vi "Autonomous Independent.vi"() -> ()   [LabVIEW 2015]
doc: "This VI is called when autonomous begins, and will automatically be terminated when autonomous ends. You can carry out timed or sensor driven robot movement independently without needing to return to the caller."
uses:
  Sprocket/src/Refname/Queues.ctl
  Auto/Auto Modes.ctl
  Sprocket/src/Action/Action Name.ctl
  Sprocket/src/Refname/Refname to String (Queue).vi
  Sprocket/src/Stream/Push Stream.vi
  Sprocket/src/Stream/Release Stream.vi
  Sprocket/lib/Sprocket.lvlib
panel:
  in  "Wedge Drop Power":dbl=0.75
  # "Be sure to right-click and choose Data Operations>>Make Current Value default if you want to save the array values with the VI"
  # "WEDGE"
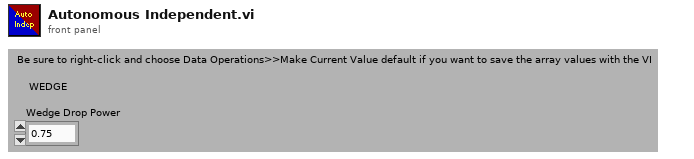
[diagram p1: front panel]
types:
  T1 = typedef "Sprocket.lvlib/Queues.ctl" = enum16{"Input", "Drive", "Collector", "Shifter", "Wedge"}
  T2 = typedef "Auto Modes.ctl" = enum16{"Do Nothing", "Drive Forward", "Cross Low Bar and Stop", "Cross Defense, No Collector", "Cross Ramparts", "Cross Low Bar, Drive to Low Goal, Shoot", "Lower Wedge, Cross Portcullis", "Back n' Forth", "Forward Spin"}
  T3 = typedef "Sprocket.lvlib/Action Name.ctl" = enum16{"No Action", "Drive Train Both", "Drive Train Rotate", "Drive Train Throttle", "Collector Motor Roll", "Collector Motor Eject", "Collector Motor Collect", "Collector Motor Stop", "Collector Extend", "Collector Retract", "Shifter High", "Shifter Low", "Collector Motor Stall", "Wedge Roll"}
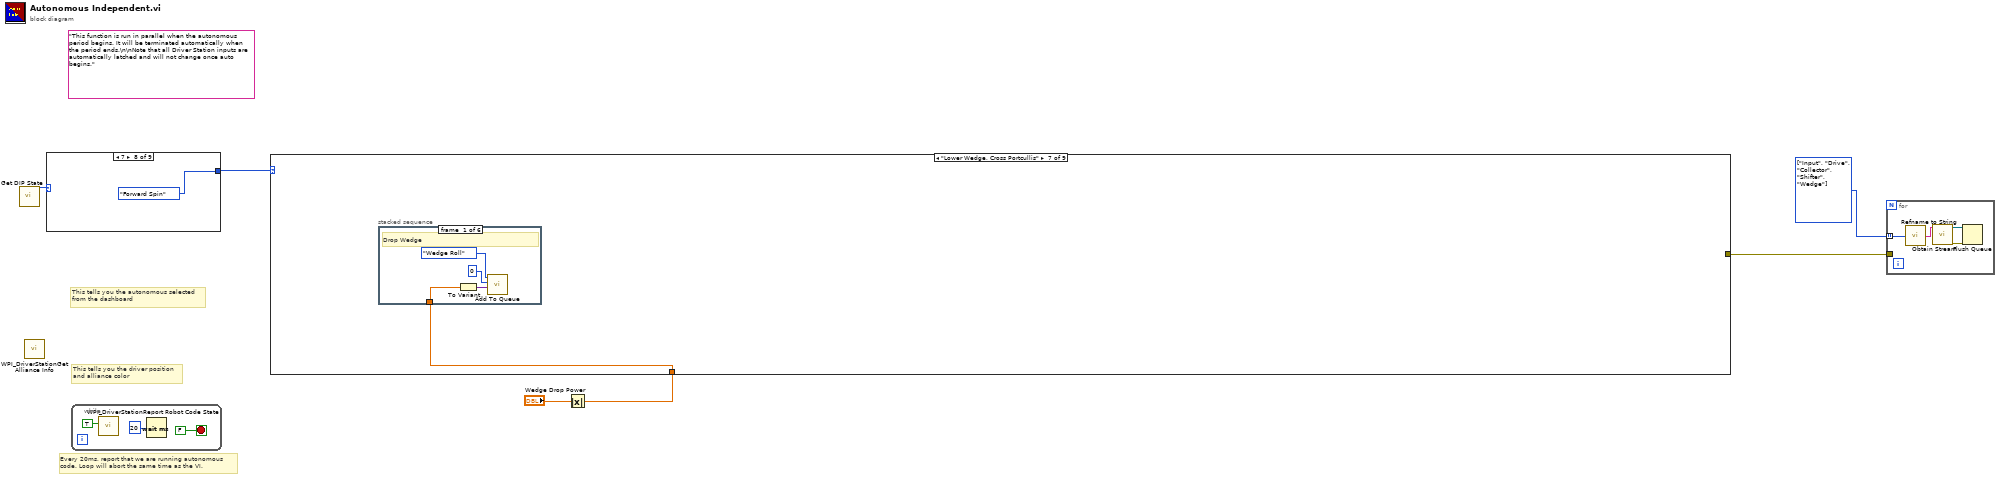
[diagram p0: block diagram]
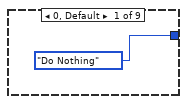
[diagram p2: hidden frame]
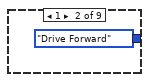
[diagram p3: hidden frame]
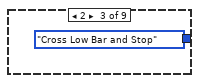
[diagram p4: hidden frame]
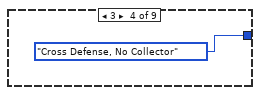
[diagram p5: hidden frame]
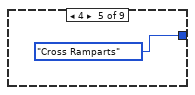
[diagram p6: hidden frame]
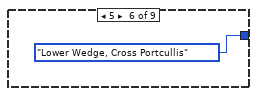
[diagram p7: hidden frame]
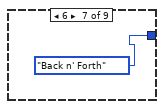
[diagram p8: hidden frame]
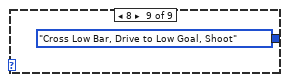
[diagram p9: hidden frame]
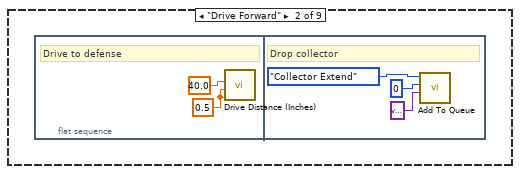
[diagram p11: hidden frame]
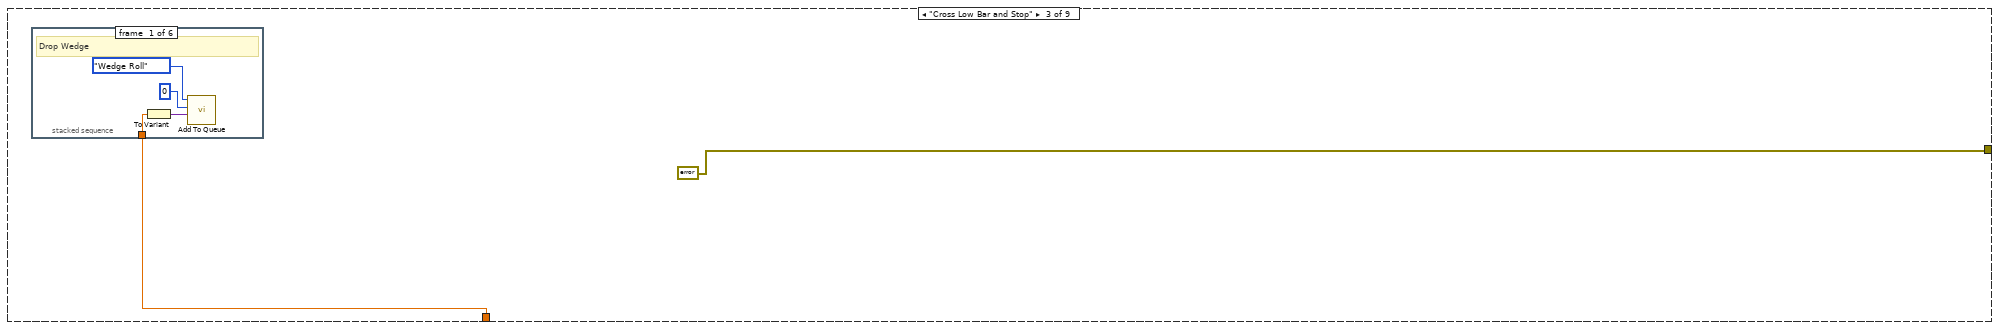
[diagram p12: hidden frame]
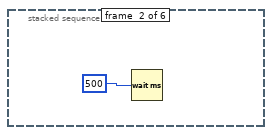
[diagram p13: hidden frame]
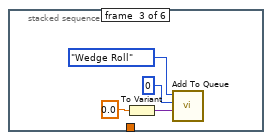
[diagram p14: hidden frame]
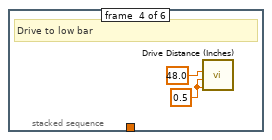
[diagram p15: hidden frame]
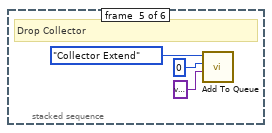
[diagram p16: hidden frame]
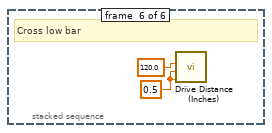
[diagram p17: hidden frame]
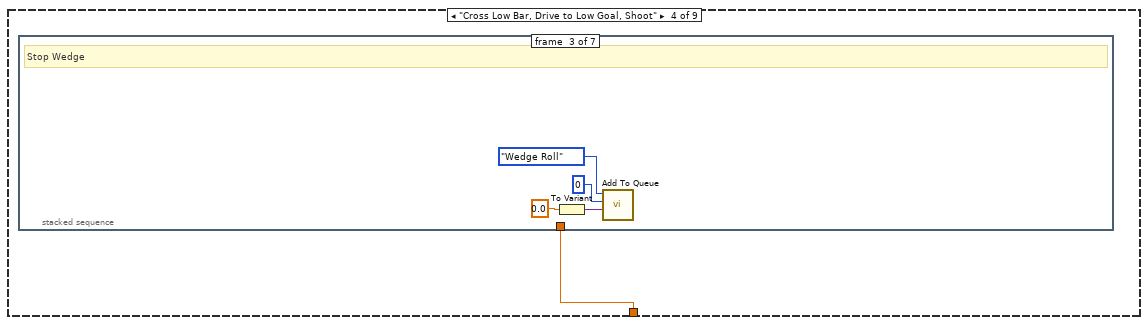
[diagram p18: hidden frame]
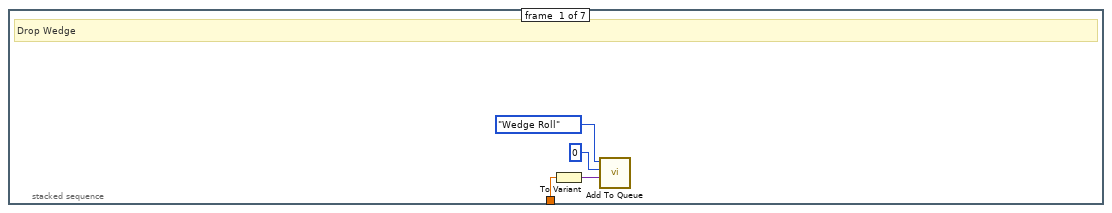
[diagram p19: hidden frame]
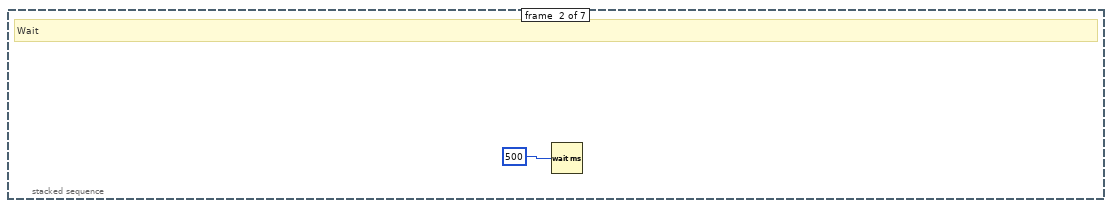
[diagram p20: hidden frame]
diagram:
  w4 = T1[] [enum."Input", enum."Drive", enum."Collector", enum."Shifter", enum."Wedge"] items=["Input", "Drive", "Collector", "Shifter", "Wedge"]
  (unwired) "This function is run in parallel when the autonomous period begins. It will be terminated automatically when the period ends.\n\nNote that all Driver Station inputs are automatically latched and will not change once auto begins."
  # "This tells you the autonomous selected\nfrom the dashboard"
  # "Every 20ms, report that we are running autonomous\ncode. Loop will abort the same time as the VI."
  # "This tells you the driver position\nand alliance color"
  n1 = call "Get DIP State.vi"() -> ("DIP State"=w5:u32)  [unwired: 10 in, 1 out]
  n2 = call <vilib>:"WPI_DriverStationGet Alliance Info.vi"() -> ()  [unwired: 12 out]
  n3 = case shown="7" w5 {
    tunnel: [Auto_Modes."Do Nothing" ("AutoModes") Auto_Modes."Drive Forward" ("AutoModes") Auto_Modes."Cross Low Bar and Stop" ("AutoModes") Auto_Modes."Cross Defense, No Collector" ("AutoModes") Auto_Modes."Cross Ramparts" ("AutoModes") Auto_Modes."Lower Wedge, Cross Portcullis" ("AutoModes") Auto_Modes."Back n' Forth" ("AutoModes") Auto_Modes."Forward Spin" ("AutoModes") Auto_Modes."Cross Low Bar, Drive to Low Goal, Shoot" ("AutoModes")] -> w6
    frame 0, Default {
    }
    frame 1 {
    }
    frame 2 {
    }
    frame 3 {
    }
    frame 4 {
    }
    frame 5 {
    }
    frame 6 {
    }
    frame 7 {
    }
    frame 8 {
    }
  }
  n4 = while {
    stop <- FALSE stop-if-true
    n5 = call <vilib>:"WPI_DriverStationReport Robot Code State.vi"("Autonomous"=TRUE) -> ()  [unwired: 10 in, 1 out]
    n6 = Wait (ms)(milliseconds to wait=u32 20) -> ()  [unwired: 1 out]
  }
  n7 = Absolute Value(x="Wedge Drop Power") -> (abs(x)=w2:dbl)
  n8 = case shown="\"Lower Wedge, Cross Portcullis\"" w6 {
    tunnel: [_ _ errorcluster {"status"=FALSE, "code"=0, "source"=""} ("error constant") _ _ _ _ _ _] -> w3
    tunnel: w2 -> [_ _ w24 w42 _ _ w74 _ _]
    frame "Do Nothing", Default {
    }
    frame "Drive Forward" {
      n9 = flat-sequence {
        frame #0 {
          w20 = 0.5 ("inches")
          # "Drive to defense"
          n10 = call "Drive Distance (Inches).vi"("Right Speed"=w20, "Left Speed"=w20, "inches"=40.0) -> ()  [unwired: 9 in]
        }
        frame #1 {
          # "Drop collector"
          n11 = call "Add To Queue.vi"("Data"=variant, "Priority"=0, "Action"=Action_Name."Collector Extend") -> ()  [unwired: 8 in, 1 out]
        }
      }
    }
    frame "Cross Low Bar and Stop" {
      n12 = stacked-sequence {
        tunnel: w24 -> [w26 _ _ _ _ _]
        frame #0 {
          # "Drop Wedge"
          n13 = To Variant(anything=w26) -> (Variant=w27:variant)
          n14 = call "Add To Queue.vi"("Data"=w27, "Priority"=0, "Action"=Action_Name."Wedge Roll") -> ()  [unwired: 8 in, 1 out]
        }
        frame #1 {
          n15 = Wait (ms)(milliseconds to wait=u32 500) -> ()  [unwired: 1 out]
        }
        frame #2 {
          n16 = To Variant(anything=0.0) -> (Variant=w32:variant)
          n17 = call "Add To Queue.vi"("Data"=w32, "Priority"=0, "Action"=Action_Name."Wedge Roll") -> ()  [unwired: 8 in, 1 out]
        }
        frame #3 {
          w35 = 0.5 ("inches")
          # "Drive to low bar"
          n18 = call "Drive Distance (Inches).vi"("Right Speed"=w35, "Left Speed"=w35, "inches"=48.0) -> ()  [unwired: 9 in]
        }
        frame #4 {
          # "Drop Collector"
          n19 = call "Add To Queue.vi"("Data"=variant, "Priority"=0, "Action"=Action_Name."Collector Extend") -> ()  [unwired: 8 in, 1 out]
        }
        frame #5 {
          w40 = 0.5 ("inches")
          # "Cross low bar"
          n20 = call "Drive Distance (Inches).vi"("Right Speed"=w40, "Left Speed"=w40, "inches"=120.0) -> ()  [unwired: 9 in]
        }
      }
    }
    frame "Cross Low Bar, Drive to Low Goal, Shoot" {
      n21 = stacked-sequence {
        tunnel: w42 -> [w43 _ _ _ _ _ _]
        frame #0 {
          # "Drop Wedge"
          n22 = To Variant(anything=w43) -> (Variant=w44:variant)
          n23 = call "Add To Queue.vi"("Data"=w44, "Priority"=0, "Action"=Action_Name."Wedge Roll") -> ()  [unwired: 8 in, 1 out]
        }
        frame #1 {
          # "Wait"
          n24 = Wait (ms)(milliseconds to wait=u32 500) -> ()  [unwired: 1 out]
        }
        frame #2 {
          # "Stop Wedge"
          n25 = To Variant(anything=0.0) -> (Variant=w49:variant)
          n26 = call "Add To Queue.vi"("Data"=w49, "Priority"=0, "Action"=Action_Name."Wedge Roll") -> ()  [unwired: 8 in, 1 out]
        }
        frame #3 {
          w52 = 0.5 ("inches")
          # "Drive to low bar"
          n27 = call "Drive Distance (Inches).vi"("Right Speed"=w52, "Left Speed"=w52, "inches"=48.0) -> ()  [unwired: 9 in]
        }
        frame #4 {
          # "Drop Collector"
          n28 = call "Add To Queue.vi"("Data"=variant, "Priority"=0, "Action"=Action_Name."Collector Extend") -> ()  [unwired: 8 in, 1 out]
        }
        frame #5 {
          w57 = 0.5 ("inches")
          # "Cross low bar"
          n29 = call "Drive Distance (Inches).vi"("Right Speed"=w57, "Left Speed"=w57, "inches"=120.0) -> ()  [unwired: 9 in]
        }
        frame #6 {
          n30 = flat-sequence {
            frame #0 {
              # "Rotate towards batter"
              n31 = call "Rotate PID.vi"("Degrees"=-120.0) -> ()  [unwired: 11 in]
            }
            frame #1 {
              # "Drive to batters"
              n32 = Negate(x=0.5) -> (-x=w62:dbl)
              n33 = call "Drive Distance (Inches).vi"("Right Speed"=w62, "Left Speed"=w62, "inches"=83.0) -> ()  [unwired: 9 in]
            }
            frame #2 {
              # "Shoot"
              n34 = Wait (ms)(milliseconds to wait=u32 500) -> ()  [unwired: 1 out]
              n35 = call "Add To Queue.vi"("Data"=variant, "Priority"=0, "Action"=Action_Name."Collector Motor Eject") -> ()  [unwired: 8 in, 1 out]
            }
            frame #3 {
              # "Stop collector"
              n36 = call "Add To Queue.vi"("Data"=variant, "Priority"=0, "Action"=Action_Name."Collector Motor Stop") -> ()  [unwired: 8 in, 1 out]
            }
          }
        }
      }
    }
    frame "Cross Defense, No Collector" {
      n37 = flat-sequence {
        frame #0 {
          w70 = 0.5 ("inches")
          # "Drive over defense"
          n38 = call "Drive Distance (Inches).vi"("Right Speed"=w70, "Left Speed"=w70, "inches"=168.0) -> ()  [unwired: 9 in]
        }
      }
    }
    frame "Cross Ramparts" {
      n39 = flat-sequence {
        frame #0 {
          w72 = 0.7 ("inches")
          # "Drive over defense"
          n40 = call "Drive Distance (Inches).vi"("Right Speed"=w72, "Left Speed"=w72, "inches"=168.0) -> ()  [unwired: 9 in]
        }
      }
    }
    frame "Lower Wedge, Cross Portcullis" {
      n41 = stacked-sequence {
        tunnel: w74 -> [w75 _ _ _ _ _]
        frame #0 {
          # "Drop Wedge"
          n42 = To Variant(anything=w75) -> (Variant=w76:variant)
          n43 = call "Add To Queue.vi"("Data"=w76, "Priority"=0, "Action"=Action_Name."Wedge Roll") -> ()  [unwired: 8 in, 1 out]
        }
        frame #1 {
          n44 = Wait (ms)(milliseconds to wait=u32 500) -> ()  [unwired: 1 out]
        }
        frame #2 {
          n45 = To Variant(anything=0.0) -> (Variant=w81:variant)
          n46 = call "Add To Queue.vi"("Data"=w81, "Priority"=0, "Action"=Action_Name."Wedge Roll") -> ()  [unwired: 8 in, 1 out]
        }
        frame #3 {
          w84 = 0.5 ("inches")
          # "Drive to low bar"
          n47 = call "Drive Distance (Inches).vi"("Right Speed"=w84, "Left Speed"=w84, "inches"=48.0) -> ()  [unwired: 9 in]
        }
        frame #4 {
          # "Drop Collector"
          n48 = call "Add To Queue.vi"("Data"=variant, "Priority"=0, "Action"=Action_Name."Collector Extend") -> ()  [unwired: 8 in, 1 out]
        }
        frame #5 {
          w89 = 0.5 ("inches")
          # "Cross low bar"
          n49 = call "Drive Distance (Inches).vi"("Right Speed"=w89, "Left Speed"=w89, "inches"=120.0) -> ()  [unwired: 9 in]
        }
      }
    }
    frame "Back n' Forth" {
    }
    frame "Forward Spin" {
      n50 = flat-sequence {
        frame #0 {
          w91 = 0.5 ("inches")
          # "Drive to Defense"
          n51 = call "Drive Distance (Inches).vi"("Right Speed"=w91, "Left Speed"=w91, "inches"=48.0) -> ()  [unwired: 9 in]
        }
        frame #1 {
          # "Drop Collector"
          n52 = call "Add To Queue.vi"("Data"=variant, "Priority"=0, "Action"=Action_Name."Collector Extend") -> ()  [unwired: 8 in, 1 out]
        }
        frame #2 {
          w96 = 0.5 ("inches")
          # "Cross Defense"
          n53 = call "Drive Distance (Inches).vi"("Right Speed"=w96, "Left Speed"=w96, "inches"=120.0) -> ()  [unwired: 9 in]
        }
        frame #3 {
          # "Spin 180"
          n54 = call "Rotate PID.vi"("Degrees"=180.0 ("Degrees to rotate 2")) -> ()  [unwired: 11 in]
        }
      }
    }
  }
  n55 = for {
    tunnel: w4 -> [w101] mode=indexing
    tunnel: w3 -> [_]
    n56 = call-poly "Refname to String.vi"("Queue Refname"=w101) -> ("Refnum Name"=w102:string)
    n57 = call "Obtain Stream.vi"("Name"=w102) -> ("error out"=w100:errorcluster, "stream out"=w99:refnum<queue>)  [unwired: 9 in]
    n58 = Flush Queue(queue=w99, error in (no error)=w100) -> ()  [unwired: 3 out]
  }
